vi "HB_ReadAIAllChannels.vi"(8 "error in (no error)":errorcluster, 11 "HBDeviceRef":T1) -> (0 "error out":errorcluster, 1 "All Channels Raw Values":u32[](array[numeric]) format="%012b", 2 "All Channels Scaled Values":dbl[](array[numeric]), 3 "HBDeviceRef":T1)   [LabVIEW 2018]
doc: "Reads all eight AI channels on the Huskie Board and returns the current values both scaled and raw."
uses:
  <vilib>/Rock Robotics/WPI/SerialPort/WPI_SerialPortRef.ctl
  <vilib>/Utility/error.llb/Error Cluster From Error Code.vi
  <vilib>/ErrorRing/Error Ring.xnode
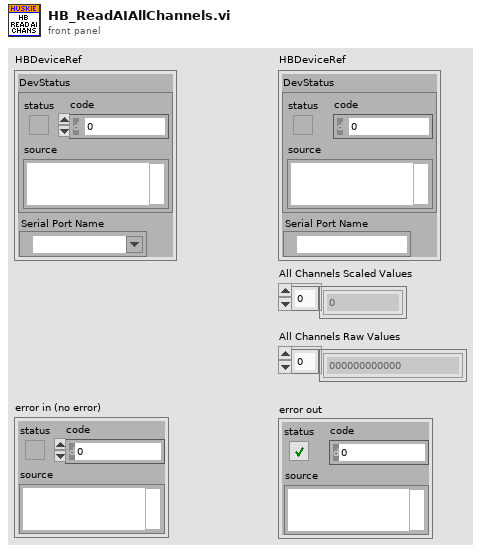
[diagram p1: front panel]
types:
  T1 = typedef "WPI_SerialPortRef.ctl" = cluster{"DevStatus":errorcluster, "Serial Port Name":refnum<visa-resource-name>}
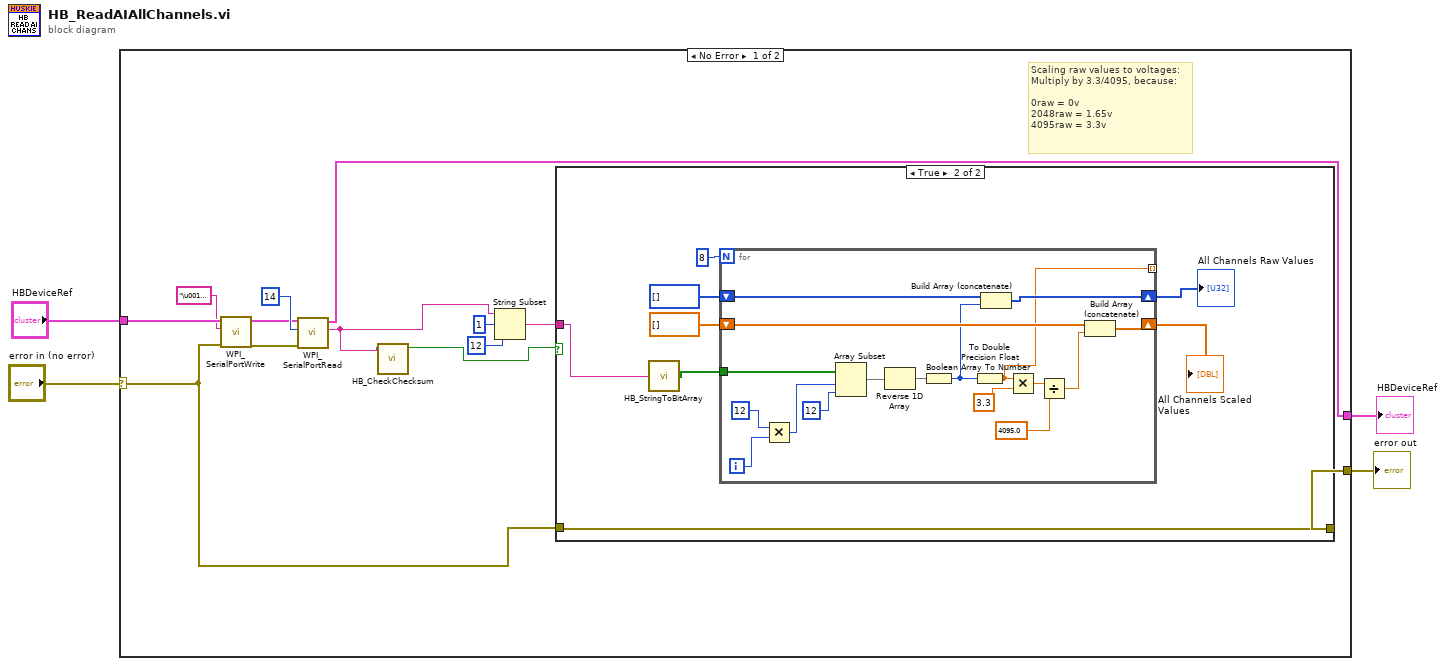
[diagram p0: block diagram]
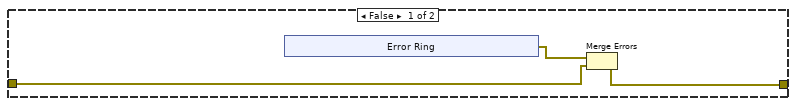
[diagram p2: hidden frame]
diagram:
  n1 = case shown="No Error" "error in (no error)" {
    selector: "error in (no error)" -> [w5 w50]
    tunnel: [w17 w50] -> w4
    tunnel: "HBDeviceRef" -> [w16 w51]
    tunnel: [w15 w51] -> w2
    frame No Error {
      # "Scaling raw values to voltages:\nMultiply by 3.3/4095, because:\n\n0raw = 0v\n2048raw = 1.65v\n4095raw = 3.3v"
      n2 = call <vilib>:"WPI_SerialPortWrite.vi"("error in (no error)"=w5, "Buffer"="\u0012\u0012", "SerialPortRef"=w16) -> ("error out"=w13:errorcluster, "SerialPortRef"=w12:T1)  [unwired: 6 in, 1 out]
      n3 = call <vilib>:"WPI_SerialPortRead.vi"("error in (no error)"=w13, "Num Bytes to Read"=u32 14, "SerialPortRef"=w12) -> ("Buffer"=w7:string, "SerialPortRef"=w15:T1)  [unwired: 6 in, 1 out]
      n4 = call <vilib>:"HB_CheckChecksum.vi"("String"=w7) -> ("Checksum Matches"=w6:bool)  [unwired: 9 in, 1 out]
      n5 = String Subset(string=w7, offset (0)=1, length (rest)=12 ("length (rest)")) -> (substring=w11:string)
      n6 = case shown="True" w6 {
        tunnel: w11 -> [_ w26]
        tunnel: w5 -> [w20 w32]
        tunnel: [w19 w32] -> w17
        frame False {
          n7 = xnode "Error Ring"() -> ("error out"=w18:errorcluster)
          n8 = Merge Errors(w18, w20) -> (w19:errorcluster)
        }
        frame True {
          n9 = call <vilib>:"HB_StringToBitArray.vi"("String"=w26) -> ("Bit Array"=w25:bool[])
          n10 = for {
            N: 8 -> [_]
            tunnel: w25 -> [w49]
            shift-right: [w45] -> w29
            shift-left: u32[] [] -> [w44]
            shift-right: [w40] -> w27
            shift-left: dbl[] [] -> [w39]
            tunnel: [w33] -> _ mode=indexing
            i -> [w48]
            n11 = Multiply(x=12, y=w48) -> (x*y=w46:i32)
            n12 = Array Subset(array=w49, index=w46, length=12) -> (w42:bool[])
            n13 = Reverse 1D Array(array=w42) -> (reversed array=w41:bool[])
            n14 = Boolean Array To Number(Boolean array=w41) -> (number=w34:u32)
            n15 = To Double Precision Float(number=w34) -> (double precision float=w33:dbl)
            n16 = Build Array (concatenate)(w44, w34) -> (w45:u32[])
            n17 = Multiply(x=w33, y=3.3) -> (x*y=w37:dbl)
            n18 = Divide(x=w37, y=4095.0) -> (x/y=w35:dbl)
            n19 = Build Array (concatenate)(w39, w35) -> (w40:dbl[])
          }
          "All Channels Raw Values" <- w29
          "All Channels Scaled Values" <- w27
        }
      }
    }
    frame Error {
    }
  }
  "error out" <- w4
  "HBDeviceRef" <- w2
